vi "SCLN_ExampleServer.vi"() -> ()   [LabVIEW 2015]
panel:
  in  "Rel2":bool
  in  "Rel1":bool
  out "Conn2":bool
  out "Conn1":bool
  out "Loop2":i32
  out "Loop1":i32
  out "Message In 2":string
  out "Message Out 2":string
  out "error out":errorcluster={"status"=TRUE, "code"=7, "source"="Open Config Data.vi"}
  in  "Config filename":path=path "/ulx1/work/devel/SCLN/config/examples.cfg"
  in  "stop":bool
  out "Message Out":string
  out "Message In":string
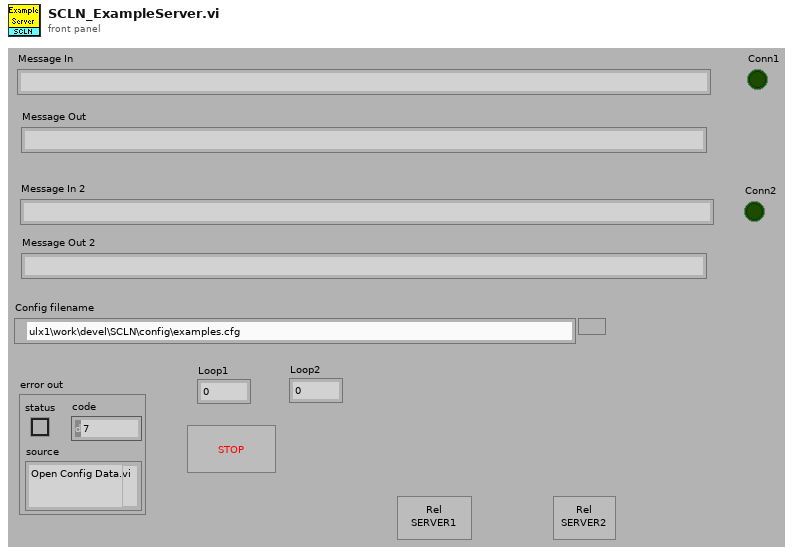
[diagram p1: front panel]
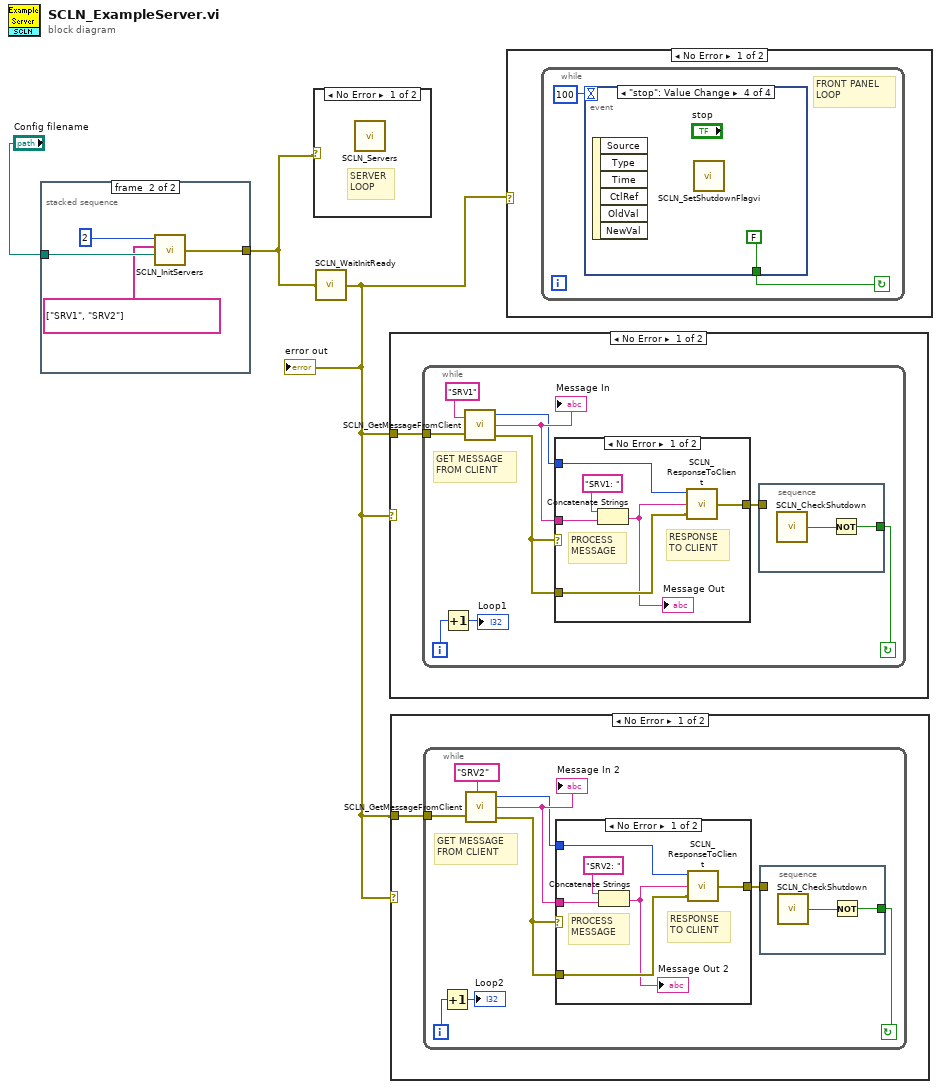
[diagram p0: block diagram]
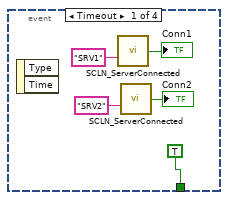
[diagram p6: hidden frame]
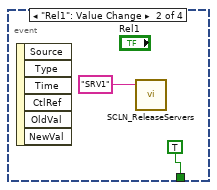
[diagram p7: hidden frame]
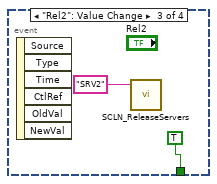
[diagram p8: hidden frame]
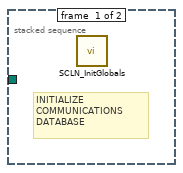
[diagram p11: hidden frame]
diagram:
  n1 = stacked-sequence {
    tunnel: "Config filename" -> [_ w6]
    tunnel: [_ w5] -> w2
    frame #0 {
      # "INITIALIZE\nCOMMUNICATIONS\nDATABASE"
      n2 = call "SCLN_InitGlobals.vi"() -> ()  [unwired: 1 in]
    }
    frame #1 {
      n3 = call "SCLN_InitServers.vi"("Config File Name"=w6, "Server Names"=string[] ["SRV1", "SRV2"], "Num of Servers"=2) -> ("error out"=w5:errorcluster)  [unwired: 1 in]
    }
  }
  n4 = case shown="No Error" w2 {
    frame No Error {
      # "SERVER\nLOOP"
      n5 = call "SCLN_Servers.vi"() -> ()  [unwired: 1 out]
    }
    frame Error {
    }
  }
  n6 = call "SCLN_WaitInitReady.vi"("error in (no error)"=w2) -> ("error out"=w1:errorcluster)
  "error out" <- w1
  n7 = case shown="No Error" w1 {
    tunnel: w1 -> [w8 _]
    frame No Error {
      n8 = while {
        tunnel: w8 -> [w17]
        i -> [w10]
        stop <- w12 continue-if-true
        # "GET MESSAGE\nFROM CLIENT"
        n9 = Increment(x=w10) -> (x+1=→"Loop1":i32)
        n10 = call "SCLN_GetMessageFromClient.vi"("Server Name"="SRV1", "error in (no error)"=w17) -> ("Index for Response"=w15:i32, "Message"=w16:string, "error out"=w14:errorcluster)
        "Message In" <- w16
        n11 = case shown="No Error" w14 {
          tunnel: w16 -> [w24 _]
          tunnel: w15 -> [w23 _]
          tunnel: w14 -> [w22 w26]
          tunnel: [w20 w26] -> w13
          frame No Error {
            # "PROCESS\nMESSAGE"
            # "RESPONSE\nTO CLIENT"
            n12 = Concatenate Strings("SRV1: ", w24) -> (w21:string)
            "Message Out" <- w21
            n13 = call "SCLN_ResponseToClient.vi"("error in (no error)"=w22, "Message"=w21, "Index for Response"=w23) -> ("error out"=w20:errorcluster)
          }
          frame Error {
          }
        }
        n14 = stacked-sequence {
          tunnel: [w18] -> w12
          tunnel: w13 -> [_]
          frame #0 {
            n15 = call "SCLN_CheckShutdown.vi"() -> ("Shutdown"=w19:bool)
            n16 = Not(x=w19) -> (.not. x?=w18:bool)
          }
        }
      }
    }
    frame Error {
    }
  }
  n17 = case shown="No Error" w1 {
    tunnel: w1 -> [w27 _]
    frame No Error {
      n18 = while {
        tunnel: w27 -> [w35]
        i -> [w28]
        stop <- w30 continue-if-true
        # "GET MESSAGE\nFROM CLIENT"
        n19 = Increment(x=w28) -> (x+1=→"Loop2":i32)
        n20 = call "SCLN_GetMessageFromClient.vi"("Server Name"="SRV2", "error in (no error)"=w35) -> ("Index for Response"=w33:i32, "Message"=w34:string, "error out"=w32:errorcluster)
        "Message In 2" <- w34
        n21 = case shown="No Error" w32 {
          tunnel: w34 -> [w43 _]
          tunnel: w33 -> [w42 _]
          tunnel: w32 -> [w41 w45]
          tunnel: [w39 w45] -> w31
          frame No Error {
            # "PROCESS\nMESSAGE"
            # "RESPONSE\nTO CLIENT"
            n22 = Concatenate Strings("SRV2: ", w43) -> (w40:string)
            "Message Out 2" <- w40
            n23 = call "SCLN_ResponseToClient.vi"("error in (no error)"=w41, "Message"=w40, "Index for Response"=w42) -> ("error out"=w39:errorcluster)
          }
          frame Error {
          }
        }
        n24 = stacked-sequence {
          tunnel: [w37] -> w30
          tunnel: w31 -> [_]
          frame #0 {
            n25 = call "SCLN_CheckShutdown.vi"() -> ("Shutdown"=w38:bool)
            n26 = Not(x=w38) -> (.not. x?=w37:bool)
          }
        }
      }
    }
    frame Error {
    }
  }
  n27 = case shown="No Error" w1 {
    frame No Error {
      n28 = while {
        stop <- w46 continue-if-true
        # "FRONT PANEL\nLOOP"
        n29 = event shown="[3] \"stop\": Value Change" {
          selector: _ -> [_ _ _ _]
          dyn-events: _ -> [_ _ _ _]
          timeout: 100 -> [_ _ _ _]
          tunnel: [TRUE TRUE TRUE FALSE] -> w46
          event Timeout {
            n30 = event-data() -> ()  [unwired: 1 in, 2 out]
            n31 = call "SCLN_ServerConnected.vi"("Server Name"="SRV1") -> ("Connected"=→"Conn1":bool)
            n32 = call "SCLN_ServerConnected.vi"("Server Name"="SRV2") -> ("Connected"=→"Conn2":bool)
          }
          event "Rel1": Value Change {
            n33 = event-data() -> ()  [unwired: 1 in, 6 out]
            n34 = call "SCLN_ReleaseServers.vi"("Server Name"="SRV1") -> ()  [unwired: 5 in]
          }
          event "Rel2": Value Change {
            n35 = event-data() -> ()  [unwired: 1 in, 6 out]
            n36 = call "SCLN_ReleaseServers.vi"("Server Name"="SRV2") -> ()  [unwired: 5 in]
          }
          event "stop": Value Change {
            n37 = event-data() -> ()  [unwired: 1 in, 6 out]
            n38 = call "SCLN_SetShutdownFlagvi.vi"() -> ()  [unwired: 1 in]
          }
        }
      }
    }
    frame Error {
    }
  }
